vi "StartIpmTrajectory.vi"(4 "error in (no error)":errorcluster, 5 "array for PVT values (max. 64 values)":T1(array[cluster]), 6 "IPM buffer parameter":T2, 7 "axis in":cluster{"keyHandle":u32, "nodeId":u16}={"keyHandle"=0, "nodeId"=1}) -> (0 "error out":errorcluster, 3 "axis out":cluster{"keyHandle":u32, "nodeId":u16}={"keyHandle"=0, "nodeId"=1})   [LabVIEW 2019, in "maxonEPOS.lvlib"]
doc: "<B>StartIpmTrajectory</B> starts the IPM trajectory with a list of PVT values."
uses:
  Examples/maxonEPOS.lvlib
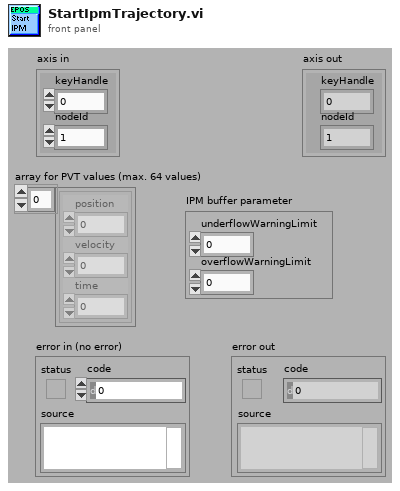
[diagram p1: front panel]
types:
  T1 = cluster{"position":i32, "velocity":i32, "time":u8}[]
  T2 = cluster{"underflowWarningLimit":u16, "overflowWarningLimit":u16}
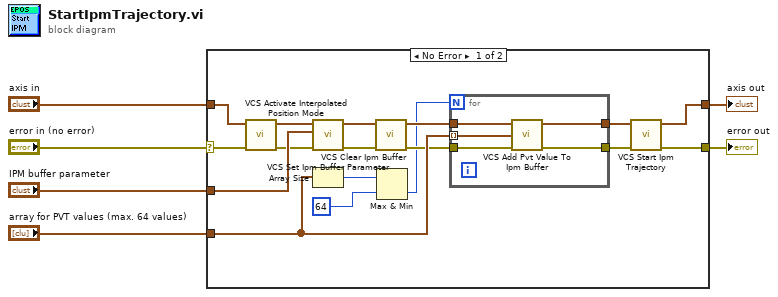
[diagram p0: block diagram]
diagram:
  n1 = case shown="No Error" "error in (no error)" {
    selector: "error in (no error)" -> [w15 w30]
    tunnel: [w22 w30] -> w5
    tunnel: [w23 w29] -> w4
    tunnel: "axis in" -> [w16 w29]
    tunnel: "IPM buffer parameter" -> [w21 _]
    tunnel: "array for PVT values (max. 64 values)" -> [w14 _]
    frame No Error {
      n2 = call "VCS Activate Interpolated Position Mode.vi"("error in (no error)"=w15, "axis in"=w16) -> ("error out"=w18:errorcluster, "axis out"=w17:cluster{"keyHandle":u32, "nodeId":u16})  [unwired: 8 in]
      n3 = call "VCS Set Ipm Buffer Parameter.vi"("error in (no error)"=w18, "IPM buffer parameter"=w21, "axis in"=w17) -> ("error out"=w19:errorcluster, "axis out"=w20:cluster{"keyHandle":u32, "nodeId":u16})  [unwired: 7 in]
      n4 = Array Size(array=w14) -> (size(s)=w9:i32)
      n5 = call "VCS Clear Ipm Buffer.vi"("error in (no error)"=w19, "axis in"=w20) -> ("error out"=w12:errorcluster, "axis out"=w13:cluster{"keyHandle":u32, "nodeId":u16})  [unwired: 8 in]
      n6 = Max & Min(x=w9, y=64) -> (min(x,y)=w8:i32)  [unwired: 1 out]
      n7 = for {
        N: w8 -> [_]
        tunnel: w14 -> [w28] mode=indexing
        tunnel: w13 -> [w27]
        tunnel: w12 -> [w26]
        tunnel: [w25] -> w11
        tunnel: [w24] -> w10
        n8 = call "VCS Add Pvt Value To Ipm Buffer.vi"("axis in"=w27, "PVT value"=w28, "error in (no error)"=w26) -> ("axis out"=w24:cluster{"keyHandle":u32, "nodeId":u16}, "error out"=w25:errorcluster)  [unwired: 11 in]
      }
      n9 = call "VCS Start Ipm Trajectory.vi"("error in (no error)"=w11, "axis in"=w10) -> ("error out"=w22:errorcluster, "axis out"=w23:cluster{"keyHandle":u32, "nodeId":u16})  [unwired: 8 in]
    }
    frame Error {
    }
  }
  "error out" <- w5
  "axis out" <- w4
